vi "MakeHTMLBody.vi"(3 "Escape Contents":bool, 4 "Body Content":string) -> (1 "Body Element":string)   [LabVIEW 2019, in "ArgosLib.lvlib"]
uses:
  ArgosLib.lvlib
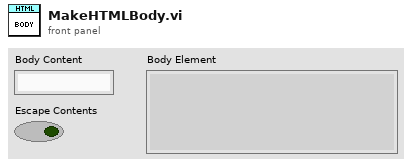
[diagram p1: front panel]
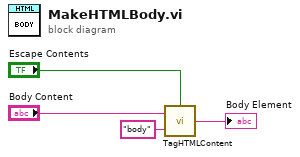
[diagram p0: block diagram]
diagram:
  n1 = call "TagHTMLContent.vi"("Escape Contents"="Escape Contents", "Tag"="body", "Element Contents"="Body Content") -> ("Tagged Contents"=→"Body Element":string)
